vi "ws Auth Save Key.vi"(8 "error in (no error)":errorcluster, 11 "Site Key":string) -> (0 "error out":errorcluster)   [LabVIEW 2011]
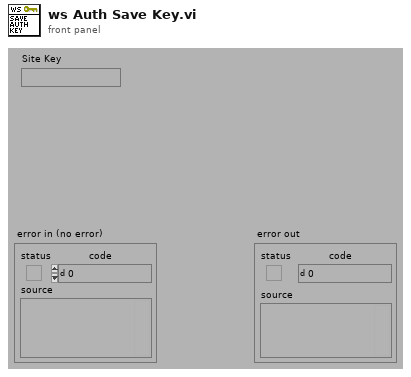
[diagram p1: front panel]
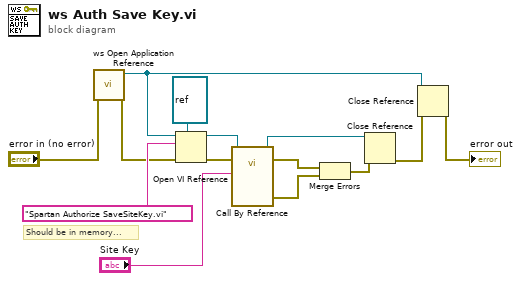
[diagram p0: block diagram]
diagram:
  # "Should be in memory..."
  n1 = call "ws Open Application Reference.vi"("error in (no error)"="error in (no error)") -> ("error out"=w1:errorcluster, "application reference"=w3:refnum<vi>)  [unwired: 9 in]
  n2 = Open VI Reference(type specifier VI Refnum (for type only)=refnum<vi> refnum, application reference (local)=w3, vi path="Spartan Authorize SaveSiteKey.vi", error in (no error)=w1) -> (vi reference=w9:refnum<vi>, error out=w10:errorcluster)  [unwired: 2 in]
  n3 = call-by-ref "?"(reference=w9, error in=w10, "Site Key Code"="Site Key") -> (reference out=w8:refnum<vi>, error out=w7:errorcluster, 0:"error out"=w6:errorcluster)  [unwired: 6 in]
  n4 = Merge Errors(w7, w6) -> (w12:errorcluster)
  n5 = Close Reference(reference=w8, error in (no error)=w12) -> (error out=w14:errorcluster)
  n6 = Close Reference(reference=w3, error in (no error)=w14) -> (error out=→"error out":errorcluster)
